vi "General Format.vi"() -> ()   [LabVIEW 2009]
panel:
  in  "VISA resource name":refnum<visa-resource-name>="GPIB0::12::INSTR"
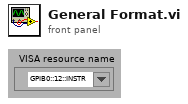
[diagram p1: front panel]
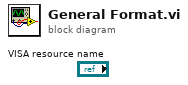
[diagram p0: block diagram]
diagram:
